vi "Project File.vi"() -> (0 "Project File":path)   [LabVIEW 2017, in "Scripts.lvlib"]
doc: "Gets the Project File (.lvproj) containg the VI."
uses:
  Scripts.lvlib
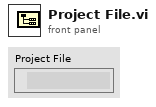
[diagram p1: front panel]
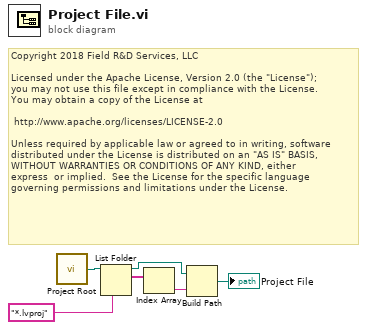
[diagram p0: block diagram]
diagram:
  # "Copyright 2018 Field R&D Services, LLC\n\nLicensed under the Apache License, Version 2.0 (the \"License\");\nyou may not use this file except in compliance with the License.\nYou may obtain a copy of the License at\n\n\thttp://www.apache.org/licenses/LICENSE-2.0\n\nUnless required by applicable law or agreed to in writing, software\ndistributed under the License is distributed on an \"AS IS\" BASIS,\nWITHOUT WARRANTIES OR CONDITIONS OF ANY KIND, either \nexpress  or implied.  See the License for the specific language \ngoverning permissions and limitations under the License."
  n1 = call "Project Root.vi"() -> ("Project Root"=w6:path)
  n2 = List Folder(path=w6, pattern="*.lvproj") -> (path out=w3:path, filenames=w4:string[])  [unwired: 2 in, 2 out]
  n3 = Index Array(array=w4) -> (element=w2:string)  [unwired: 1 in]
  n4 = Build Path(base path=w3, name or relative path=w2) -> (appended path=→"Project File":path)
